vi "TEST_GUI.vi"() -> ()   [LabVIEW 2013]
panel:
  in  "stop":bool
  in  "curent set":u16
  out "CURRENT":dbl
  out "VOLTAGE":dbl
  in  "on/off":bool
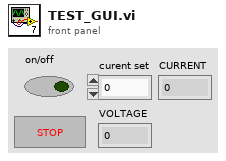
[diagram p1: front panel]
types:
  T1 = typedef "MagnetCluster.ctl" = cluster{"Main interlock":bool, "Flow Switch 1":bool, "Flow Switch 2":bool, "Power Supply ok":bool, "on":bool, "staging":bool, "undulator":bool, "VOLTAGE":dbl, "CURRENT":dbl, "curent set":u16}
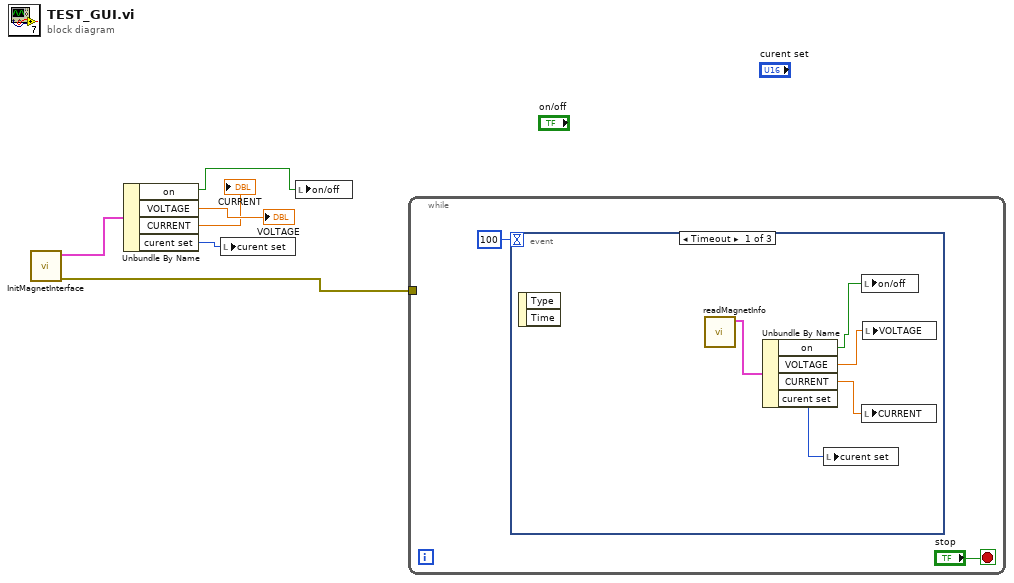
[diagram p0: block diagram]
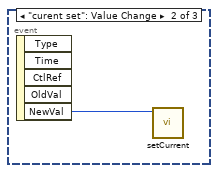
[diagram p2: hidden frame]
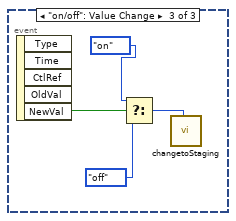
[diagram p3: hidden frame]
diagram:
  n1 = call "InitMagnetInterface.vi"() -> ("error out"=w6:errorcluster, "output cluster 2"=w1:T1)  [unwired: 10 in]
  n2 = Unbundle By Name(w1) -> ("on"=w3:bool, "VOLTAGE"=→"VOLTAGE":dbl, "CURRENT"=→"CURRENT":dbl, "curent set"=w2:u16)
  n3 = local write "curent set"(w2) -> ()
  n4 = local write "on/off"(w3) -> ()
  n5 = while {
    tunnel: w6 -> [_]
    stop <- "stop" stop-if-true
    n6 = event shown="[0] Timeout" {
      selector: _ -> [_ _ _]
      dyn-events: _ -> [_ _ _]
      timeout: 100 -> [_ _ _]
      event Timeout {
        n7 = event-data() -> ()  [unwired: 1 in, 2 out]
        n8 = call "readMagnetInfo.vi"() -> ("output cluster"=w13:T1)  [unwired: 10 in, 1 out]
        n9 = Unbundle By Name(w13) -> ("on"=w12:bool, "VOLTAGE"=w10:dbl, "CURRENT"=w11:dbl, "curent set"=w9:u16)
        n10 = local write "curent set"(w9) -> ()
        n11 = local write "on/off"(w12) -> ()
        n12 = local write "CURRENT"(w11) -> ()
        n13 = local write "VOLTAGE"(w10) -> ()
      }
      event "curent set": Value Change {
        n14 = event-data() -> ("NewVal"=w14:u16)  [unwired: 1 in, 4 out]
        n15 = call "setCurrent.vi"("curent set"=w14) -> ()  [unwired: 10 in, 1 out]
      }
      event "on/off": Value Change {
        n16 = event-data() -> ("NewVal"=w18:bool)  [unwired: 1 in, 4 out]
        n17 = Select(t=enum16{"off", "on", "undulator", "staging"}."on" ("cmd"), s=w18, f=enum16{"off", "on", "undulator", "staging"}."off" ("cmd")) -> (s? t:f=w15:enum16{"off", "on", "undulator", "staging"})
        n18 = call "changetoStaging.vi"("cmd"=w15) -> ()  [unwired: 10 in, 1 out]
      }
    }
  }
